vi "Filter Unexpired Paths.vi"(0 "Path Groups in":refnum<class "Path Group.lvclass">[](array[class]), 11 "Error in (no error)":errorcluster) -> (4 "Path Groups out":refnum<class "Path Group.lvclass">[](array[class]), 6 "Path Count":i32, 10 "Paths Filtered out":refnum<class "Path.lvclass">[](array[class]), 15 "Error out":errorcluster)   [LabVIEW 2023, in "RFCalAndFixtureCharact.Common.lvlib"]
uses:
  RFCalAndFixtureCharact.Common.lvlib
  Base Classes/Path Group/Path Group.lvclass
  Base Classes/Path/Path.lvclass
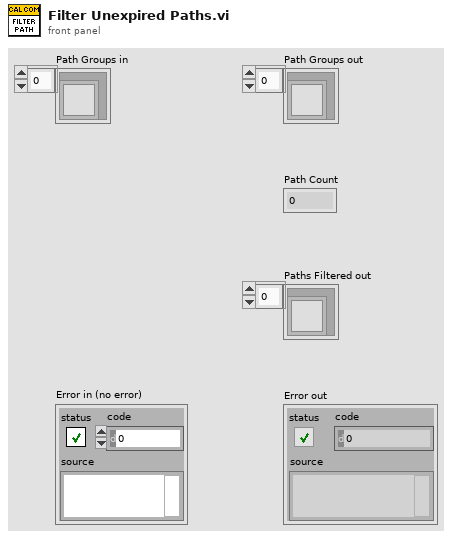
[diagram p1: front panel]
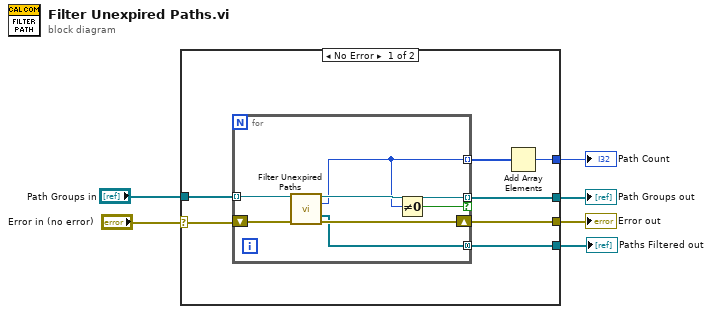
[diagram p0: block diagram]
diagram:
  n1 = case shown="No Error" "Error in (no error)" {
    selector: "Error in (no error)" -> [w13 w22]
    tunnel: [w12 w21] -> w5
    tunnel: [w11 w22] -> w4
    tunnel: [w10 _] -> w3
    tunnel: "Path Groups in" -> [w9 w21]
    tunnel: [w7 _] -> w1
    frame No Error {
      n2 = for {
        shift-right: [w19] -> w11
        shift-left: w13 -> [w20]
        tunnel: [w18] -> w12 mode=indexing if=w17
        tunnel: w9 -> [w16] mode=indexing
        tunnel: [w15] -> w8 mode=indexing
        tunnel: [w14] -> w7 mode=concatenating
        n3 = call "Filter Unexpired Paths.vi"("Path Group in"=w16, "error in (no error)"=w20) -> ("Path Group out"=w18:refnum<class "Path Group.lvclass">, "Expired Path Count"=w15:i32, "Paths Filtered out"=w14:refnum<class "Path.lvclass">[], "error out"=w19:errorcluster)  [unwired: 10 in]
        n4 = Not Equal To 0?(x=w15) -> (x != 0?=w17:bool)
      }
      n5 = Add Array Elements(numeric array=w8) -> (sum=w10:i32)
    }
    frame Error {
    }
  }
  "Error out" <- w4
  "Path Count" <- w3
  "Path Groups out" <- w5
  "Paths Filtered out" <- w1
